vi "PM5000_PQ_THD.vi"(8 "error in":errorcluster, 11 "Network Path":string="172.22.26.202") -> (0 "error out":errorcluster, 1 "THD_array":sgl[](array[numeric]), 2 "THD_cluster":T1, 3 "Network Path out":string="192.168.169.1")   [LabVIEW 2018]
doc: "Lee la tabla de memoria RealTime_VIF_Power del equipo PowerMonitor 5000, ademas filtra y ordena las variables de interez de la tabla de memoria.\n\nLee las siguientes variables de la tabla RealTime_VIF_Power:\n\n*V1_V2_Volts\n*V2_V3_Volts\n*V3_V1_Volts\n*I1_Amps\n*I2_Amps\n*I3_Amps\n*Frequency_Hz\n*Total_kW\n*Total_kVAR\n*Total_kVA\n*Total_True_PF\n*Total_Disp_PF"
uses:
  Controls/THD_cluster.ctl
  <vilib>/ethernetip/ethernetip.llb/EthernetIP SLC500 Read Float.vi
  <vilib>/ethernetip/ethernetip.lvlib
panel:
  out "V_unbalance_%":sgl
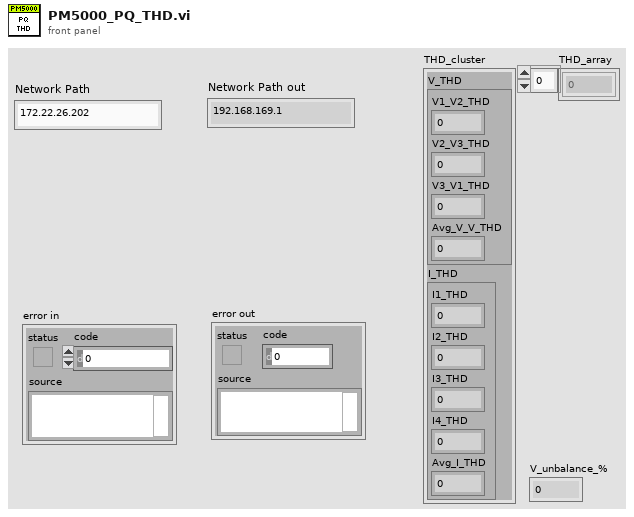
[diagram p1: front panel]
types:
  T1 = typedef "THD_cluster.ctl" = cluster{"V_THD":cluster{"V1_V2_THD":sgl, "V2_V3_THD":sgl, "V3_V1_THD":sgl, "Avg_V_V_THD":sgl}, "I_THD":cluster{"I1_THD":sgl, "I2_THD":sgl, "I3_THD":sgl, "I4_THD":sgl, "Avg_I_THD":sgl}}
  T2 = cluster{"V1_V2_THD":sgl, "V2_V3_THD":sgl, "V3_V1_THD":sgl, "Avg_V_V_THD":sgl}
  T3 = cluster{"I1_THD":sgl, "I2_THD":sgl, "I3_THD":sgl, "I4_THD":sgl, "Avg_I_THD":sgl}
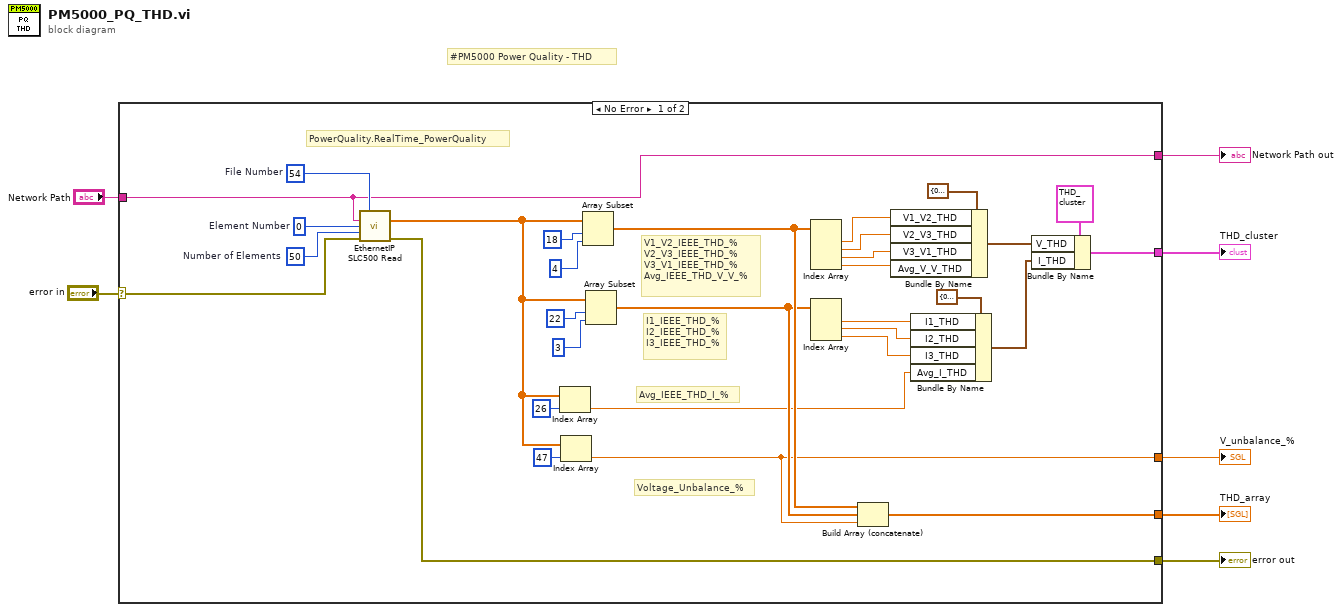
[diagram p0: block diagram]
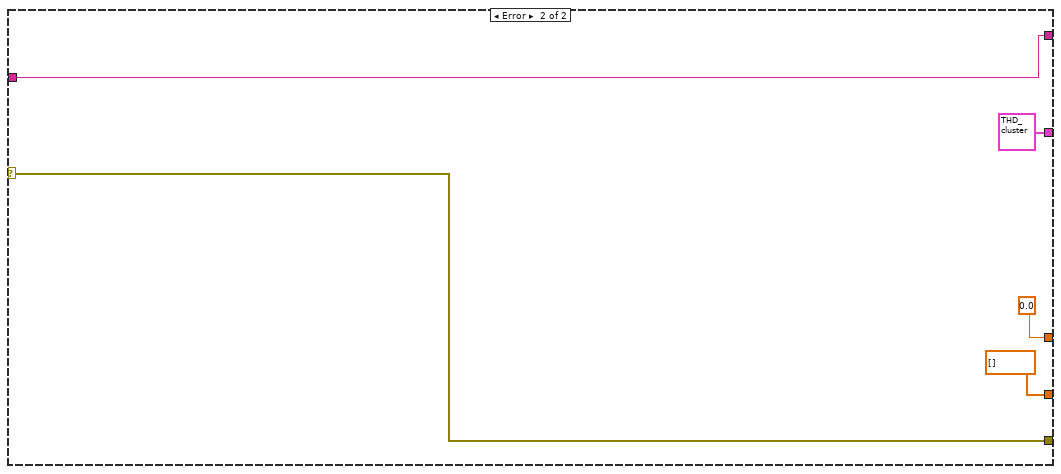
[diagram p2: hidden frame]
diagram:
  # "#PM5000 Power Quality - THD"
  n1 = case shown="No Error" "error in" {
    selector: "error in" -> [w30 w43]
    tunnel: [w35 w43] -> w7
    tunnel: [w19 w42] -> w5
    tunnel: [w20 T1 {"V_THD"={"V1_V2_THD"=0.0, "V2_V3_THD"=0.0, "V3_V1_THD"=0.0, "Avg_V_V_THD"=0.0}, "I_THD"={"I1_THD"=0.0, "I2_THD"=0.0, "I3_THD"=0.0, "I4_THD"=0.0, "Avg_I_THD"=0.0}} ("THD_cluster")] -> w3
    tunnel: "Network Path" -> [w19 w42]
    tunnel: [w16 sgl 0.0] -> w2
    tunnel: [w15 sgl[] []] -> w1
    frame No Error {
      w36 = u32 50  # Number of Elements
      w38 = u16 54  # File Number
      w37 = u16 0  # Element Number
      # "Avg_IEEE_THD_I_%"
      # "Voltage_Unbalance_%"
      # "I1_IEEE_THD_%\nI2_IEEE_THD_%\nI3_IEEE_THD_%"
      # "V1_V2_IEEE_THD_%\nV2_V3_IEEE_THD_%\nV3_V1_IEEE_THD_%\nAvg_IEEE_THD_V_V_%"
      # "PowerQuality.RealTime_PowerQuality"
      n2 = call-poly <vilib>:"EthernetIP SLC500 Read.vi"("File Number"=w38, "Network Path"=w19, "Element Number"=w37, "Number of Elements"=w36, "error in"=w30) -> ("Data"=w14:sgl[], "error out"=w35:errorcluster)  [unwired: 8 in, 1 out]
      n3 = Index Array(array=w14, index=26) -> (element=w12:sgl)
      n4 = Index Array(array=w14, index=47) -> (element=w16:sgl)
      n5 = Array Subset(array=w14, index=18, length=4) -> (w18:sgl[])
      n6 = Array Subset(array=w14, index=22, length=3) -> (w17:sgl[])
      n7 = Index Array(array=w18) -> (element #1=w28:sgl, element #2=w27:sgl, element #3=w26:sgl, element #4=w25:sgl)  [unwired: 4 in]
      n8 = Index Array(array=w17) -> (element #1=w24:sgl, element #2=w23:sgl, element #3=w22:sgl)  [unwired: 3 in]
      n9 = Build Array (concatenate)(w18, w17, w16) -> (w15:sgl[])
      n10 = Bundle By Name(cluster=T2 {"V1_V2_THD"=0.0, "V2_V3_THD"=0.0, "V3_V1_THD"=0.0, "Avg_V_V_THD"=0.0} ("V_THD"), "V1_V2_THD"=w28, "V2_V3_THD"=w27, "V3_V1_THD"=w26, "Avg_V_V_THD"=w25) -> (w9:T2)
      n11 = Bundle By Name(cluster=T3 {"I1_THD"=0.0, "I2_THD"=0.0, "I3_THD"=0.0, "I4_THD"=0.0, "Avg_I_THD"=0.0} ("I_THD"), "I1_THD"=w24, "I2_THD"=w23, "I3_THD"=w22, "Avg_I_THD"=w12) -> (w8:T3)
      n12 = Bundle By Name(cluster=T1 {"V_THD"={"V1_V2_THD"=0.0, "V2_V3_THD"=0.0, "V3_V1_THD"=0.0, "Avg_V_V_THD"=0.0}, "I_THD"={"I1_THD"=0.0, "I2_THD"=0.0, "I3_THD"=0.0, "I4_THD"=0.0, "Avg_I_THD"=0.0}} ("THD_cluster"), "V_THD"=w9, "I_THD"=w8) -> (w20:T1)
    }
    frame Error {
    }
  }
  "error out" <- w7
  "Network Path out" <- w5
  "THD_cluster" <- w3
  "V_unbalance_%" <- w2
  "THD_array" <- w1
